vi "MenuAction.vi"(8 "error in (no error)":errorcluster caption="错误输入（无错误）", 10 "项标识符":string, 11 "TrendPlot 输入":refnum<class "TrendPlot.lvclass">) -> (0 "error out":errorcluster caption="错误输出", 3 "TrendPlot 输出":refnum<class "TrendPlot.lvclass">)   [LabVIEW 2018, in "DataDisplay.lvlib" / "TrendPlot.lvclass"]
uses:
  TrendPlot.lvclass
  TrendPlot.lvclass/TrendPlot.ctl
  TypeDefine/DD_Command.ctl
  DataDisplay.lvlib
panel:
  out "selected path":path
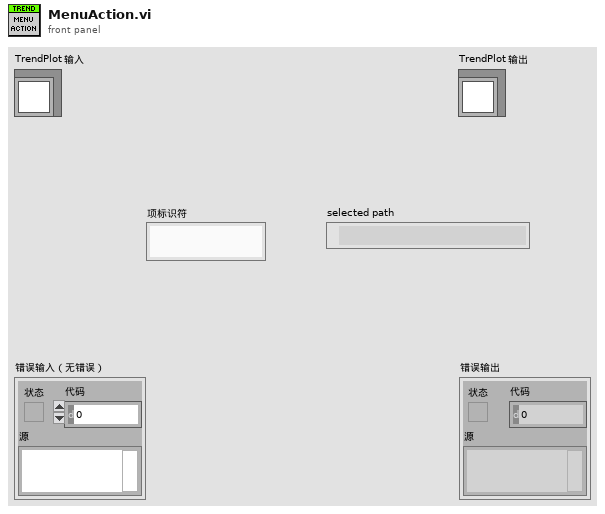
[diagram p1: front panel]
types:
  T1 = typedef "DataDisplay.lvlib/DD_Command.ctl" = cluster{"消息":string, "参数":variant}
  T2 = typedef "imagedata.ctl" = cluster{"image type":i32, "image depth":i32, "image":u8[], "mask":u8[], "colors":u32[], "Rectangle":cluster{"left":i16, "top":i16, "right":i16, "bottom":i16}}
  T3 = typedef "DataDisplay.lvlib/DD_CommandQ.ctl" = refnum<queue>
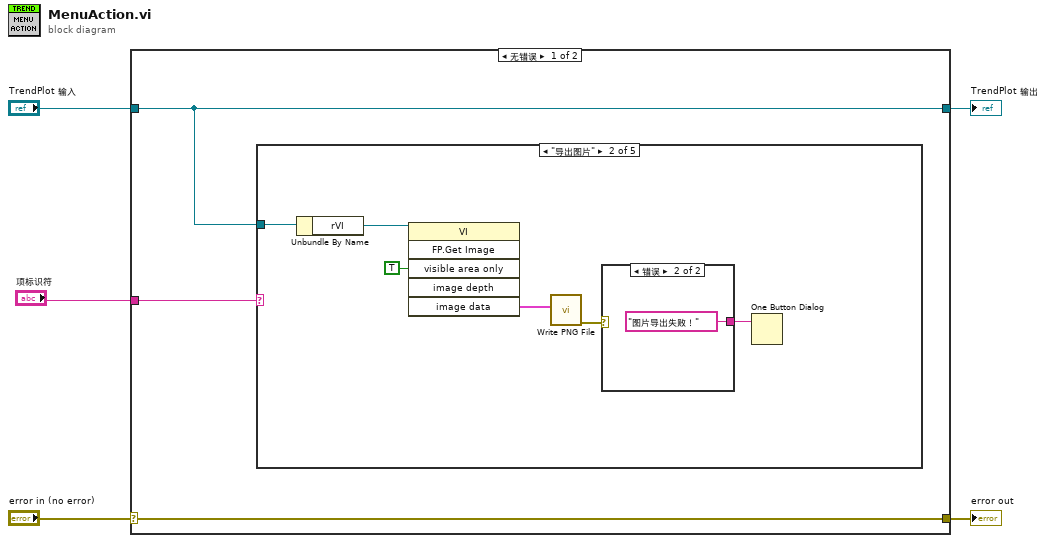
[diagram p0: block diagram]
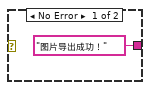
[diagram p3: hidden frame]
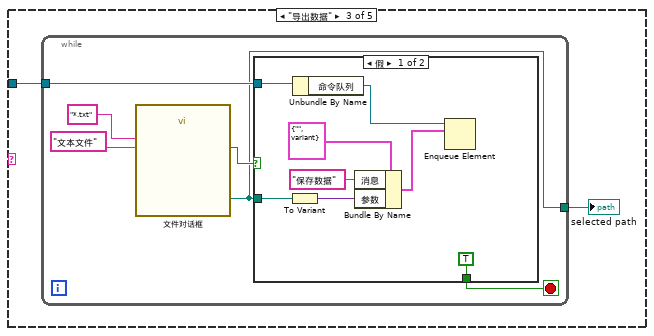
[diagram p4: hidden frame]
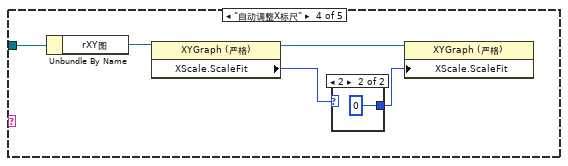
[diagram p6: hidden frame]
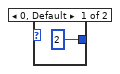
[diagram p7: hidden frame]
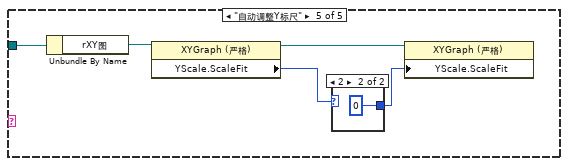
[diagram p8: hidden frame]
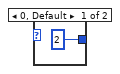
[diagram p9: hidden frame]
diagram:
  n1 = case shown="无错误" "error in (no error)" {
    selector: "error in (no error)" -> [w8 w49]
    tunnel: [w8 w49] -> w4
    tunnel: [w6 w48] -> w2
    tunnel: "TrendPlot 输入" -> [w6 w48]
    tunnel: "项标识符" -> [w7 _]
    frame No Error {
      n2 = case shown="\"导出图片\"" w7 {
        tunnel: w6 -> [_ w14 w17 w38 w45]
        frame "假", Default {
        }
        frame "导出图片" {
          n3 = Unbundle By Name(w14) -> ("rVI"=w13:refnum<vi>)
          n4 = invoke class="VI" method="FP.Get Image"(reference=w13, "visible area only"=TRUE ("仅可见区域")) -> ("image data"=w12:T2)  [unwired: 4 in, 5 out]
          n5 = call <vilib>:"Write PNG File.vi"("image data"=w12) -> ("error out"=w10:errorcluster)  [unwired: 9 in, 1 out]
          n6 = case shown="错误" w10 {
            tunnel: ["图片导出成功！" "图片导出失败！"] -> w9
            frame No Error {
            }
            frame Error {
            }
          }
          n7 = One Button Dialog(message=w9) -> ()  [unwired: 1 in, 1 out]
        }
        frame "导出数据" {
          n8 = while {
            tunnel: [w19] -> w18
            tunnel: w17 -> [w20]
            stop <- w21 stop-if-true
            n9 = call "文件对话框"("pattern (all files)"="*.txt", "pattern label"="文本文件") -> ("selected path"=w19:path, "cancelled"=w22:bool)  [unwired: 10 in, 2 out]
            n10 = case shown="假" w22 {
              selector: w22 -> [_ w33]
              tunnel: [TRUE w33] -> w21
              tunnel: w20 -> [w31 _]
              tunnel: w19 -> [w27 _]
              frame False {
                n11 = To Variant(anything=w27) -> (Variant=w26:variant)
                n12 = Unbundle By Name(w31) -> ("命令队列"=w30:T3)
                n13 = Bundle By Name(cluster=T1 {"消息"="", "参数"=variant} ("元素"), "消息"="保存数据", "参数"=w26) -> (w25:T1)
                n14 = Enqueue Element(queue=w30, element=w25) -> ()  [unwired: 2 in, 3 out]
              }
              frame True {
              }
            }
          }
          "selected path" <- w18
        }
        frame "自动调整X标尺" {
          n15 = Unbundle By Name(w38) -> ("rXY图"=w37:refnum<vi>)
          n16 = property class="XYGraph (严格)"(reference=w37) -> (reference out=w35:refnum<vi>, "XScale.ScaleFit"=w36:u8)  [unwired: 1 in, 1 out]
          n17 = case shown="2" w36 {
            tunnel: [u8 2 ("X标尺.标尺调节") u8 0 ("X标尺.标尺调节")] -> w34
            frame 0, Default {
            }
            frame 2 {
            }
          }
          n18 = property class="XYGraph (严格)"(reference=w35, "XScale.ScaleFit"=w34) -> ()  [unwired: 1 in, 2 out]
        }
        frame "自动调整Y标尺" {
          n19 = Unbundle By Name(w45) -> ("rXY图"=w44:refnum<vi>)
          n20 = property class="XYGraph (严格)"(reference=w44) -> (reference out=w42:refnum<vi>, "YScale.ScaleFit"=w43:u8)  [unwired: 1 in, 1 out]
          n21 = case shown="2" w43 {
            tunnel: [u8 2 ("X标尺.标尺调节") u8 0 ("X标尺.标尺调节")] -> w41
            frame 0, Default {
            }
            frame 2 {
            }
          }
          n22 = property class="XYGraph (严格)"(reference=w42, "YScale.ScaleFit"=w41) -> ()  [unwired: 1 in, 2 out]
        }
      }
    }
    frame Error {
    }
  }
  "error out" <- w4
  "TrendPlot 输出" <- w2
